vi "ConnectToPub.vi"(3 "LogPath in":path, 4 "ROS":T2, 5 "IP":string) -> (0 "LogPath out":path, 1 "Log":T1, 2 "PubRef":refnum<k5>)   [LabVIEW 2014]
doc: "Connect subscriber to publisher"
uses:
  <userlib>/ROS for LabVIEW Software.lnk/ROS/Code/SubVIs/_ROSControl.ctl
  <userlib>/ROS for LabVIEW Software.lnk/ROS/Code/SubVIs/_ROSDirection.ctl
  <userlib>/ROS for LabVIEW Software.lnk/ROS/Code/Console/Servers/ServerSubs/ROSLog.ctl
  <userlib>/ROS for LabVIEW Software.lnk/ROS/Code/Console/Servers/ServerSubs/MyState.ctl
  <userlib>/ROS for LabVIEW Software.lnk/ROS/Code/_ROSDefinition.vi
panel:
  in  "error in (no error)":errorcluster
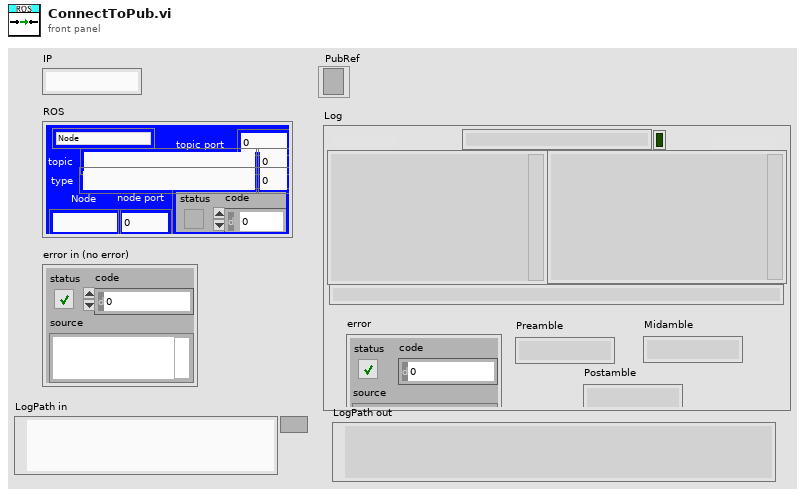
[diagram p1: front panel]
types:
  T1 = cluster{"Sent":string, "Reply":string, "MethodName":string, "success":bool, "Dir1":string, "Dir2":string, "Time Stamp":string, "error":errorcluster, "Preamble":string, "Midamble":string, "Postamble":string}
  T2 = typedef "_ROSControl.ctl" = cluster{"topic port":u16, "Node":string, "topic":string, "type":string, "node port":u16, "error ":errorcluster, "Direction":T3, "Update (ms)":u16, "FIFO size":u16}
  T3 = typedef "_ROSDirection.ctl" = enum16{"Node", "Publisher", "Subscriber", "ServiceClient", "ServiceProvider"}
  T4 = typedef "MyState.ctl" = enum16{"No Connection", "Registered", "Connected", "Close"}
  T5 = typedef "ROSLog.ctl" = cluster{"Sent":string, "Reply":string, "MethodName":string, "success":bool, "Dir1":string, "Dir2":string, "Time Stamp":string, "error":errorcluster, "Preamble":string, "Midamble":string, "Postamble":string}
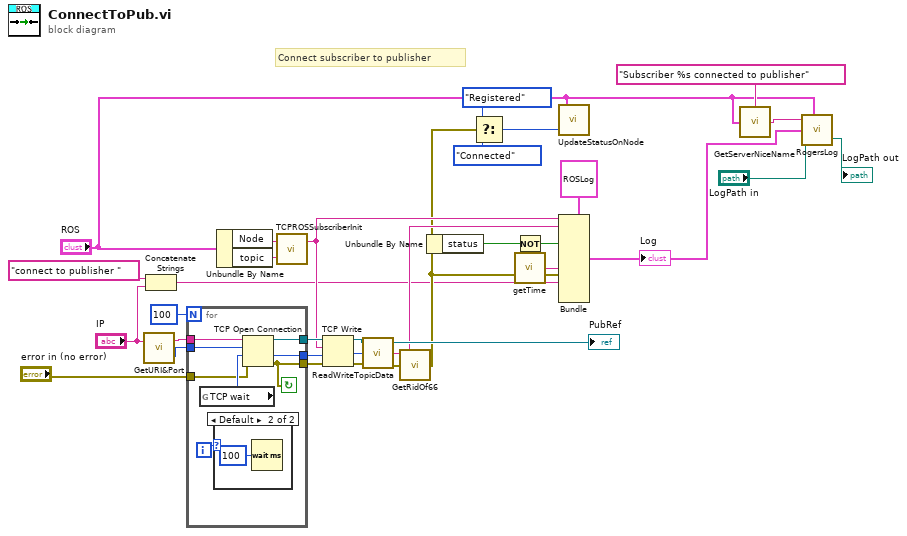
[diagram p0: block diagram]
diagram:
  # "Connect subscriber to publisher"
  n1 = call <userlib>:"GetURI&Port.vi"("URI in"="IP") -> ("Port"=w32:u16, "URI"=w31:string)
  n2 = Concatenate Strings("connect to publisher ", "IP") -> (w8:string)
  n3 = for {
    N: 100 -> [_]
    tunnel: w32 -> [w39]
    tunnel: w31 -> [w38]
    tunnel: [w37] -> w30
    tunnel: "error in (no error)" -> [w36]
    tunnel: [w33] -> w23
    tunnel: [w35] -> w22
    i -> [w34]
    stop <- w33 continue-if-true
    n4 = global read "_ROSDefinition.vi" "TCP wait"() -> (w37:i32)
    n5 = case shown="Default" w34 {
      frame 0 {
      }
      frame Default {
        n6 = Wait (ms)(milliseconds to wait=u32 100) -> ()  [unwired: 1 out]
      }
    }
    n7 = TCP Open Connection(address=w38, remote port or service name=w39, timeout ms (60000)=w37, error in (no error)=w36) -> (connection ID=w35:refnum<k5>, error out=w33:errorcluster)  [unwired: 1 in]
  }
  n8 = Unbundle By Name("ROS") -> ("Node"=w20:string, "topic"=w21:string)
  n9 = call <userlib>:"TCPROSSubscriberInit.vi"("topic"=w21, "callerID"=w20) -> ("TCP ROS Reply"=w18:string)  [unwired: 1 in]
  n10 = TCP Write(connection ID=w22, data in=w18, error in (no error)=w23, 9:w30) -> (connection ID out=w24:refnum<k5>, error out=w25:errorcluster)  [unwired: 1 out]
  n11 = call <userlib>:"ReadWriteTopicData.vi"("error in (no error)"=w25, "timeout ms (1000)"=w30, "connection ID in"=w24) -> ("error out"=w13:errorcluster, "data out"=w19:string, "connection ID out"=→"PubRef":refnum<k5>)
  n12 = call <userlib>:"GetRidOf66.vi"("error in (no error)"=w13) -> ("error out"=w12:errorcluster)
  n13 = Unbundle By Name(w12) -> ("status"=w15:bool)
  n14 = Select(t=MyState."Registered" ("MyState"), s=w12, f=MyState."Connected" ("MyState")) -> (s? t:f=w11:T4)
  n15 = Not(x=w15) -> (.not. x?=w16:bool)
  n16 = call <userlib>:"getTime.vi"() -> ("Current Time"=w17:string)  [unwired: 1 in]
  n17 = call <userlib>:"UpdateStatusOnNode.vi"("MyState"=w11, "ROS"="ROS") -> ()  [unwired: 1 in, 1 out]
  n18 = Bundle(cluster=T5 {"Sent"="", "Reply"="", "MethodName"="Publisher ID", "success"=FALSE, "Dir1"="To ROS", "Dir2"="From ROS", "Time Stamp"="", "error"={"status"=FALSE, "code"=0, "source"=""}, "Preamble"="", "Midamble"="", "Postamble"=""} ("Log"), "Sent"=w18, "Reply"=w19, "success"=w16, "Time Stamp"=w17, "error"=w12, "Preamble"=w8) -> (w4:T5)  [unwired: 5 in]
  "Log" <- w4
  n19 = call <userlib>:"GetServerNiceName.vi"("ROS"="ROS", "Text to add"="Subscriber %s connected to publisher") -> ("String"=w7:string)
  n20 = call <userlib>:"RogersLog.vi"("Text to add"=w7, "ROS"="ROS", "Log"=w4, "LogPath in"="LogPath in") -> ("LogPath out"=→"LogPath out":path)  [unwired: 1 in, 1 out]
